vi "Example -- Producer-Monitor as a Queue (FIFO).vi"() -> ()   [LabVIEW 2013]
uses:
  VariantBuffer/buffer-type -- enum.ctl
  VariantBuffer/VariantBuffer.lvclass
panel:
  out "data":string[](array[string])
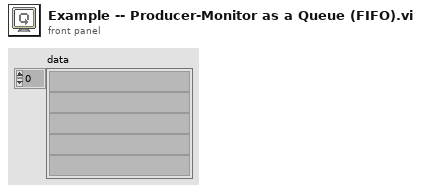
[diagram p1: front panel]
types:
  T1 = typedef "CircularBuffer.lvlib/VariantBuffer.lvclass/buffer-type -- enum.ctl" = enum16{"Queue", "Stack"}
  T2 = typedef "VariantBuffer.lvclass/buffer-event -- enum.ctl" = enum16{"element-added", "element-removed", "filled", "emptied", "resized", "default-changed", "destroyed"}
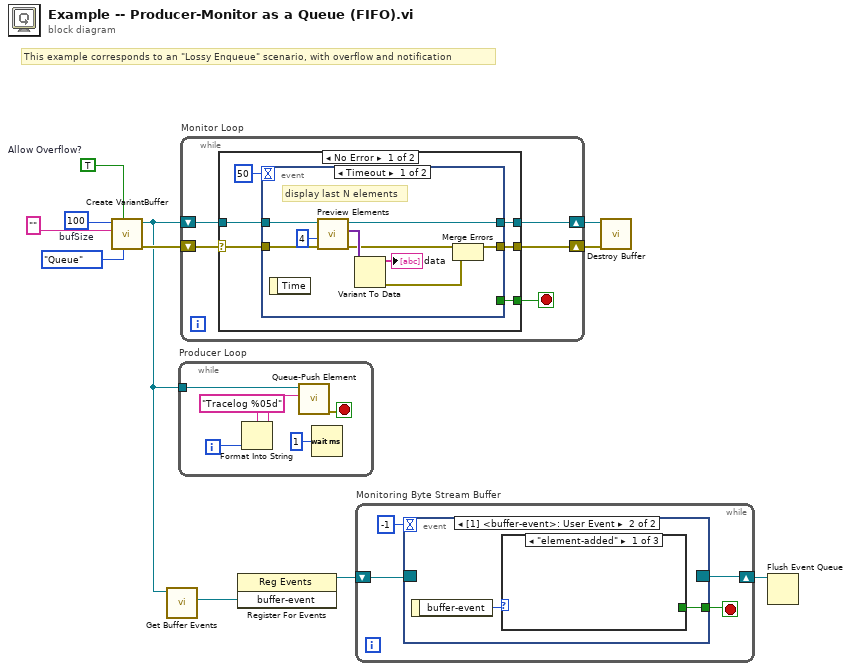
[diagram p0: block diagram]
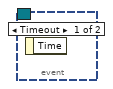
[diagram p2: hidden frame]
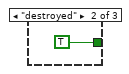
[diagram p3: hidden frame]
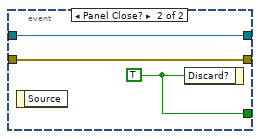
[diagram p5: hidden frame]
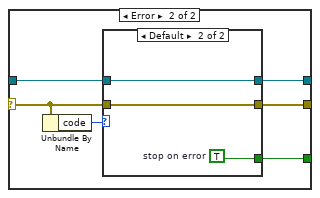
[diagram p6: hidden frame]
diagram:
  w1 = TRUE  # Allow Overflow?
  w11 = 100  # bufSize
  # "This example corresponds to an \"Lossy Enqueue\" scenario, with overflow and notification"
  n1 = call "Create VariantBuffer.vi"("buffer-type"=buffer-type_--_enum."Queue", "Allow Overflow?"=w1, "default"="", "bufSize"=w11) -> ("error out"=w8:errorcluster, "Buffer"=w3:refnum<data-value>)  [unwired: 6 in]
  n2 = call "Get Buffer Events.vi"("Buffer in"=w3) -> ("buffer-event"=w6:refnum<user-event>)  [unwired: 8 in, 2 out]
  n3 = while "Producer Loop" {
    tunnel: w3 -> [w14]
    i -> [w16]
    stop <- w12 stop-if-true
    n4 = Format Into String(format string="Tracelog %05d", w16) -> (resulting string=w13:string)  [unwired: 2 in, 1 out]
    n5 = call "Queue-Push Element.vi"("element"=w13, "Buffer in"=w14) -> ("error out"=w12:errorcluster)  [unwired: 5 in, 4 out]
    n6 = Wait (ms)(milliseconds to wait=u32 1) -> ()  [unwired: 1 out]
  }
  n7 = while "Monitor Loop" {
    shift-right: [w21] -> w9
    shift-left: w3 -> [w22]
    shift-right: [w20] -> w7
    shift-left: w8 -> [w18]
    stop <- w19 stop-if-true
    n8 = case shown="No Error" w18 {
      selector: w18 -> [w23 w42]
      tunnel: w22 -> [w27 w43]
      tunnel: [w26 w44] -> w21
      tunnel: [w25 w41] -> w20
      tunnel: [w24 w46] -> w19
      frame No Error {
        n9 = event shown="[0] Timeout" {
          selector: _ -> [_ _]
          dyn-events: _ -> [_ _]
          timeout: 50 -> [_ _]
          tunnel: w27 -> [w36 w40]
          tunnel: [w35 w40] -> w26
          tunnel: [_ w39] -> w24
          tunnel: w23 -> [w32 w38]
          tunnel: [w31 w38] -> w25
          event Timeout {
            # "display last N elements"
            n10 = event-data() -> ()  [unwired: 1 in, 1 out]
            n11 = call "Preview Elements.vi"("error in"=w32, "count (-1: all)"=4, "ByteBuffer in"=w36) -> ("error out"=w30:errorcluster, "elements"=w33:variant[], "ByteBuffer"=w35:refnum<data-value>)  [unwired: 6 in]
            n12 = Variant To Data(Variant=w33) -> (data=→"data":string[], error out=w29:errorcluster)  [unwired: 2 in]
            n13 = Merge Errors(w30, w29) -> (w31:errorcluster)
          }
          event Panel Close? {
            w39 = TRUE ("Discard?")
            n14 = event-data() -> ()  [unwired: 1 in, 1 out]
            n15 = event-data("Discard?"=w39) -> ()  [unwired: 1 in, 1 out]
          }
        }
      }
      frame Error {
        n16 = Unbundle By Name(w42) -> ("code"=w45:i32)
        n17 = case shown="Default" w45 {
          tunnel: [_ w50] -> w46
          tunnel: [w47 w49] -> w44
          tunnel: w43 -> [w47 w49]
          tunnel: w42 -> [_ w48]
          tunnel: [_ w48] -> w41
          frame 0 {
            # "Handle Error\n& Continue"
          }
          frame Default {
            w50 = TRUE  # stop on error
          }
        }
      }
    }
  }
  n18 = register-events(w6) -> (reference out=w5:refnum<event-registration>)  [unwired: 2 in, 1 out]
  n19 = while "Monitoring Byte Stream Buffer" {
    shift-right: [w52] -> w4
    shift-left: w5 -> [w53]
    stop <- w51 stop-if-true
    n20 = event shown="[1] <buffer-event>: User Event" {
      selector: w53 -> [_ _]
      dyn-events: [_ _] -> w52
      timeout: -1 -> [_ _]
      tunnel: [_ w55] -> w51
      event Timeout {
        n21 = event-data() -> ()  [unwired: 1 in, 1 out]
      }
      event User Event {
        n22 = event-data() -> ("buffer-event"=w56:T2)  [unwired: 1 in]
        n23 = case shown="\"element-added\"" w56 {
          tunnel: [_ TRUE _] -> w55
          frame "element-added" {
          }
          frame "destroyed" {
          }
          frame Default {
          }
        }
      }
    }
  }
  n24 = call "Destroy Buffer.vi"("error in"=w7, "Buffer"=w9) -> ()  [unwired: 8 in, 2 out]
  n25 = Flush Event Queue(0:w4) -> ()  [unwired: 5 in, 3 out]
